vi "decide_state.vi"(0 "state in":T1={"State"=enum."sense", "Maze"=[[FALSE, FALSE, FALSE, FALSE, FALSE, FALSE, FALSE, FALSE, FALSE], [FALSE, FALSE, TRUE, FALSE, FALSE, TRUE, TRUE, TRUE, FALSE], [FALSE, FALSE, TRUE, TRUE, TRUE, TRUE, FALSE, FALSE, FALSE], [FALSE, FALSE, TRUE, FALSE, FALSE, TRUE, FALSE, FALSE, FALSE], [TRUE, TRUE, TRUE, FALSE, FALSE, TRUE, FALSE, TRUE, TRUE], [FALSE, FALSE, FALSE, TRUE, TRUE, TRUE, FALSE, TRUE, FALSE], [FALSE, FALSE, FALSE, FALSE, FALSE, TRUE, TRUE, TRUE, FALSE], [FALSE, FALSE, FALSE, FALSE, FALSE, FALSE, FALSE, FALSE, FALSE], [FALSE, FALSE, FALSE, FALSE, FALSE, FALSE, FALSE, FALSE, FALSE]], "Runner Row"=0, "Runner Column"=0, "Runner Direction"=enum."east", "Sense"={"wall in front"=FALSE, "wall to left"=FALSE, "wall to right"=FALSE, "wall behind"=FALSE, "exit column"=FALSE}, "Hand"=enum."Left-handed"}) -> (4 "state out":T1={"State"=enum."sense", "Maze"=[[FALSE, FALSE, FALSE, FALSE, FALSE, FALSE, FALSE, FALSE, FALSE], [FALSE, FALSE, TRUE, FALSE, FALSE, TRUE, TRUE, TRUE, FALSE], [FALSE, FALSE, TRUE, TRUE, TRUE, TRUE, FALSE, FALSE, FALSE], [FALSE, FALSE, TRUE, FALSE, FALSE, TRUE, FALSE, FALSE, FALSE], [TRUE, TRUE, TRUE, FALSE, FALSE, TRUE, FALSE, TRUE, TRUE], [FALSE, FALSE, FALSE, TRUE, TRUE, TRUE, FALSE, TRUE, FALSE], [FALSE, FALSE, FALSE, FALSE, FALSE, TRUE, TRUE, TRUE, FALSE], [FALSE, FALSE, FALSE, FALSE, FALSE, FALSE, FALSE, FALSE, FALSE], [FALSE, FALSE, FALSE, FALSE, FALSE, FALSE, FALSE, FALSE, FALSE]], "Runner Row"=0, "Runner Column"=0, "Runner Direction"=enum."east", "Sense"={"wall in front"=FALSE, "wall to left"=FALSE, "wall to right"=FALSE, "wall behind"=FALSE, "exit column"=FALSE}, "Hand"=enum."Left-handed"})   [LabVIEW 2016]
uses:
  typedefs/state.ctl
  typedefs/action_start.ctl
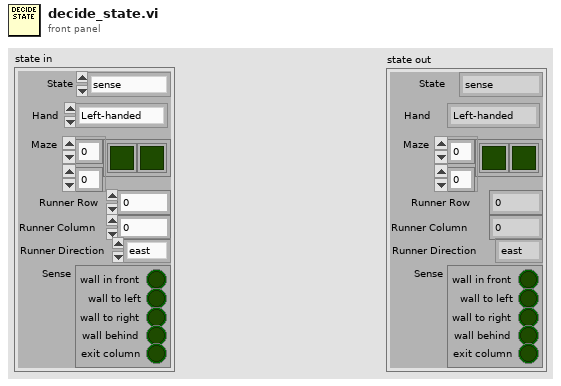
[diagram p1: front panel]
types:
  T1 = typedef "state.ctl" = cluster{"State":T2, "Maze":bool[][], "Runner Row":i32, "Runner Column":i32, "Runner Direction":enum16{"east", "north", "west", "south"}, "Sense":cluster{"wall in front":bool, "wall to left":bool, "wall to right":bool, "wall behind":bool, "exit column":bool}, "Hand":enum16{"Left-handed", "Right-handed"}}
  T2 = typedef "action_start.ctl" = enum16{"sense", "decide", "step", "pivot right", "pivot left", "stop"}
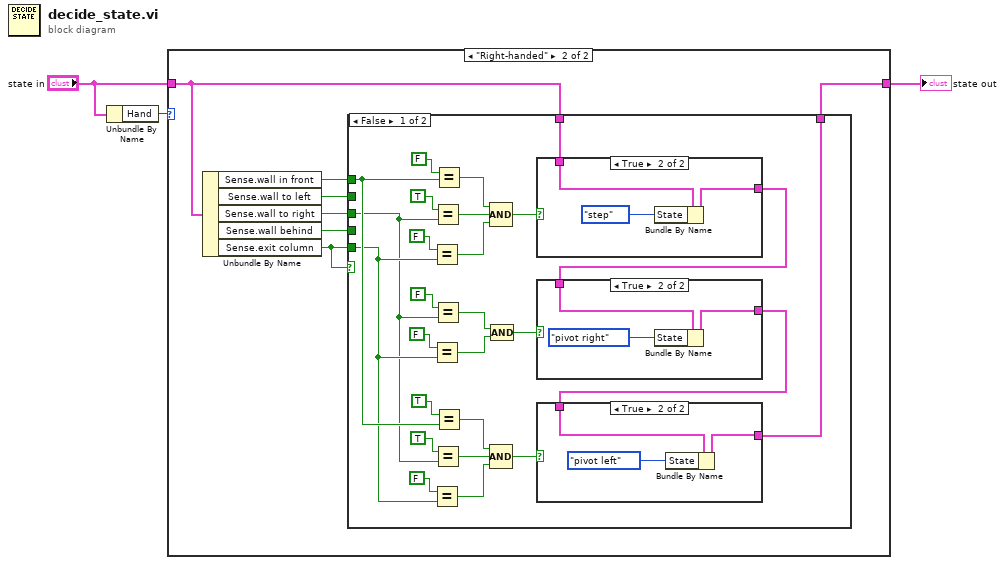
[diagram p0: block diagram]
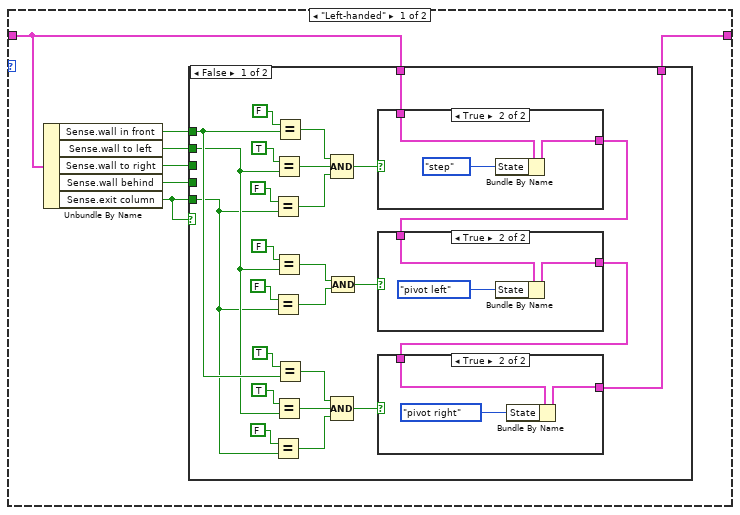
[diagram p2: hidden frame]
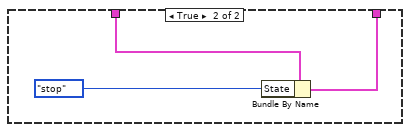
[diagram p6: hidden frame]
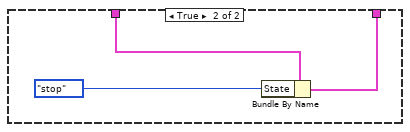
[diagram p10: hidden frame]
diagram:
  n1 = Unbundle By Name("state in") -> ("Hand"=w2:enum16{"Left-handed", "Right-handed"})
  n2 = case shown="\"Right-handed\"" w2 {
    tunnel: "state in" -> [w5 w53]
    tunnel: [w4 w52] -> w3
    frame "Left-handed" {
      n3 = Unbundle By Name(w5) -> ("Sense.wall in front"=w10:bool, "Sense.wall to left"=w9:bool, "Sense.wall to right"=w8:bool, "Sense.wall behind"=w7:bool, "Sense.exit column"=w6:bool)
      n4 = case shown="False" w6 {
        tunnel: w5 -> [w24 w51]
        tunnel: w10 -> [w16 _]
        tunnel: w9 -> [w15 _]
        tunnel: w8 -> [_ _]
        tunnel: w7 -> [_ _]
        tunnel: w6 -> [w14 _]
        tunnel: [w11 w49] -> w4
        frame False {
          n5 = Equal?(x=FALSE, y=w14) -> (x = y?=w31:bool)
          n6 = Equal?(x=FALSE, y=w14) -> (x = y?=w25:bool)
          n7 = Equal?(x=FALSE, y=w14) -> (x = y?=w22:bool)
          n8 = Equal?(x=TRUE, y=w15) -> (x = y?=w32:bool)
          n9 = Equal?(x=FALSE, y=w15) -> (x = y?=w26:bool)
          n10 = Equal?(x=TRUE, y=w15) -> (x = y?=w21:bool)
          n11 = Equal?(x=FALSE, y=w16) -> (x = y?=w33:bool)
          n12 = Equal?(x=TRUE, y=w16) -> (x = y?=w20:bool)
          n13 = Compound Arithmetic op=AND(w33, w32, w31) -> (w30:bool)
          n14 = Compound Arithmetic op=AND(w20, w21, w22) -> (w13:bool)
          n15 = Compound Arithmetic op=AND(w26, w25) -> (w27:bool)
          n16 = case shown="True" w30 {
            tunnel: w24 -> [w45 w47]
            tunnel: [w45 w46] -> w23
            frame False {
            }
            frame True {
              n17 = Bundle By Name(cluster=w47, "State"=action_start."step" ("action start")) -> (w46:T1)
            }
          }
          n18 = case shown="True" w27 {
            tunnel: w23 -> [w41 w42]
            tunnel: [w41 w43] -> w12
            frame False {
            }
            frame True {
              n19 = Bundle By Name(cluster=w42, "State"=action_start."pivot left" ("action start")) -> (w43:T1)
            }
          }
          n20 = case shown="True" w13 {
            tunnel: w12 -> [w37 w40]
            tunnel: [w37 w39] -> w11
            frame False {
            }
            frame True {
              n21 = Bundle By Name(cluster=w40, "State"=action_start."pivot right" ("action start")) -> (w39:T1)
            }
          }
        }
        frame True {
          n22 = Bundle By Name(cluster=w51, "State"=action_start."stop" ("action start")) -> (w49:T1)
        }
      }
    }
    frame "Right-handed" {
      n23 = Unbundle By Name(w53) -> ("Sense.wall in front"=w58:bool, "Sense.wall to left"=w57:bool, "Sense.wall to right"=w56:bool, "Sense.wall behind"=w55:bool, "Sense.exit column"=w54:bool)
      n24 = case shown="False" w54 {
        tunnel: w53 -> [w72 w99]
        tunnel: w58 -> [w64 _]
        tunnel: w57 -> [_ _]
        tunnel: w56 -> [w59 _]
        tunnel: w55 -> [_ _]
        tunnel: w54 -> [w63 _]
        tunnel: [w60 w97] -> w52
        frame False {
          n25 = Equal?(x=FALSE, y=w63) -> (x = y?=w79:bool)
          n26 = Equal?(x=FALSE, y=w63) -> (x = y?=w73:bool)
          n27 = Equal?(x=FALSE, y=w63) -> (x = y?=w70:bool)
          n28 = Equal?(x=TRUE, y=w59) -> (x = y?=w80:bool)
          n29 = Equal?(x=FALSE, y=w59) -> (x = y?=w74:bool)
          n30 = Equal?(x=TRUE, y=w59) -> (x = y?=w69:bool)
          n31 = Equal?(x=FALSE, y=w64) -> (x = y?=w81:bool)
          n32 = Equal?(x=TRUE, y=w64) -> (x = y?=w68:bool)
          n33 = Compound Arithmetic op=AND(w81, w80, w79) -> (w78:bool)
          n34 = Compound Arithmetic op=AND(w68, w69, w70) -> (w62:bool)
          n35 = Compound Arithmetic op=AND(w74, w73) -> (w75:bool)
          n36 = case shown="True" w78 {
            tunnel: w72 -> [w93 w95]
            tunnel: [w93 w94] -> w71
            frame False {
            }
            frame True {
              n37 = Bundle By Name(cluster=w95, "State"=action_start."step" ("action start")) -> (w94:T1)
            }
          }
          n38 = case shown="True" w75 {
            tunnel: w71 -> [w89 w90]
            tunnel: [w89 w91] -> w61
            frame False {
            }
            frame True {
              n39 = Bundle By Name(cluster=w90, "State"=action_start."pivot right" ("action start")) -> (w91:T1)
            }
          }
          n40 = case shown="True" w62 {
            tunnel: w61 -> [w85 w88]
            tunnel: [w85 w87] -> w60
            frame False {
            }
            frame True {
              n41 = Bundle By Name(cluster=w88, "State"=action_start."pivot left" ("action start")) -> (w87:T1)
            }
          }
        }
        frame True {
          n42 = Bundle By Name(cluster=w99, "State"=action_start."stop" ("action start")) -> (w97:T1)
        }
      }
    }
  }
  "state out" <- w3
